vi "insertSoc_trans.vi"(8 "error in (no error)":errorcluster, 10 "input cluster":T3, 11 "connection reference":T1) -> (0 "error out":errorcluster, 3 "connection reference out":T1)   [LabVIEW 2012]
uses:
  <vilib>/addons/database/Connection.llb/Conn ObjectReference.ctl
  <vilib>/addons/database/NI_Database_API.lvlib
panel:
  in  "Cluster":T2
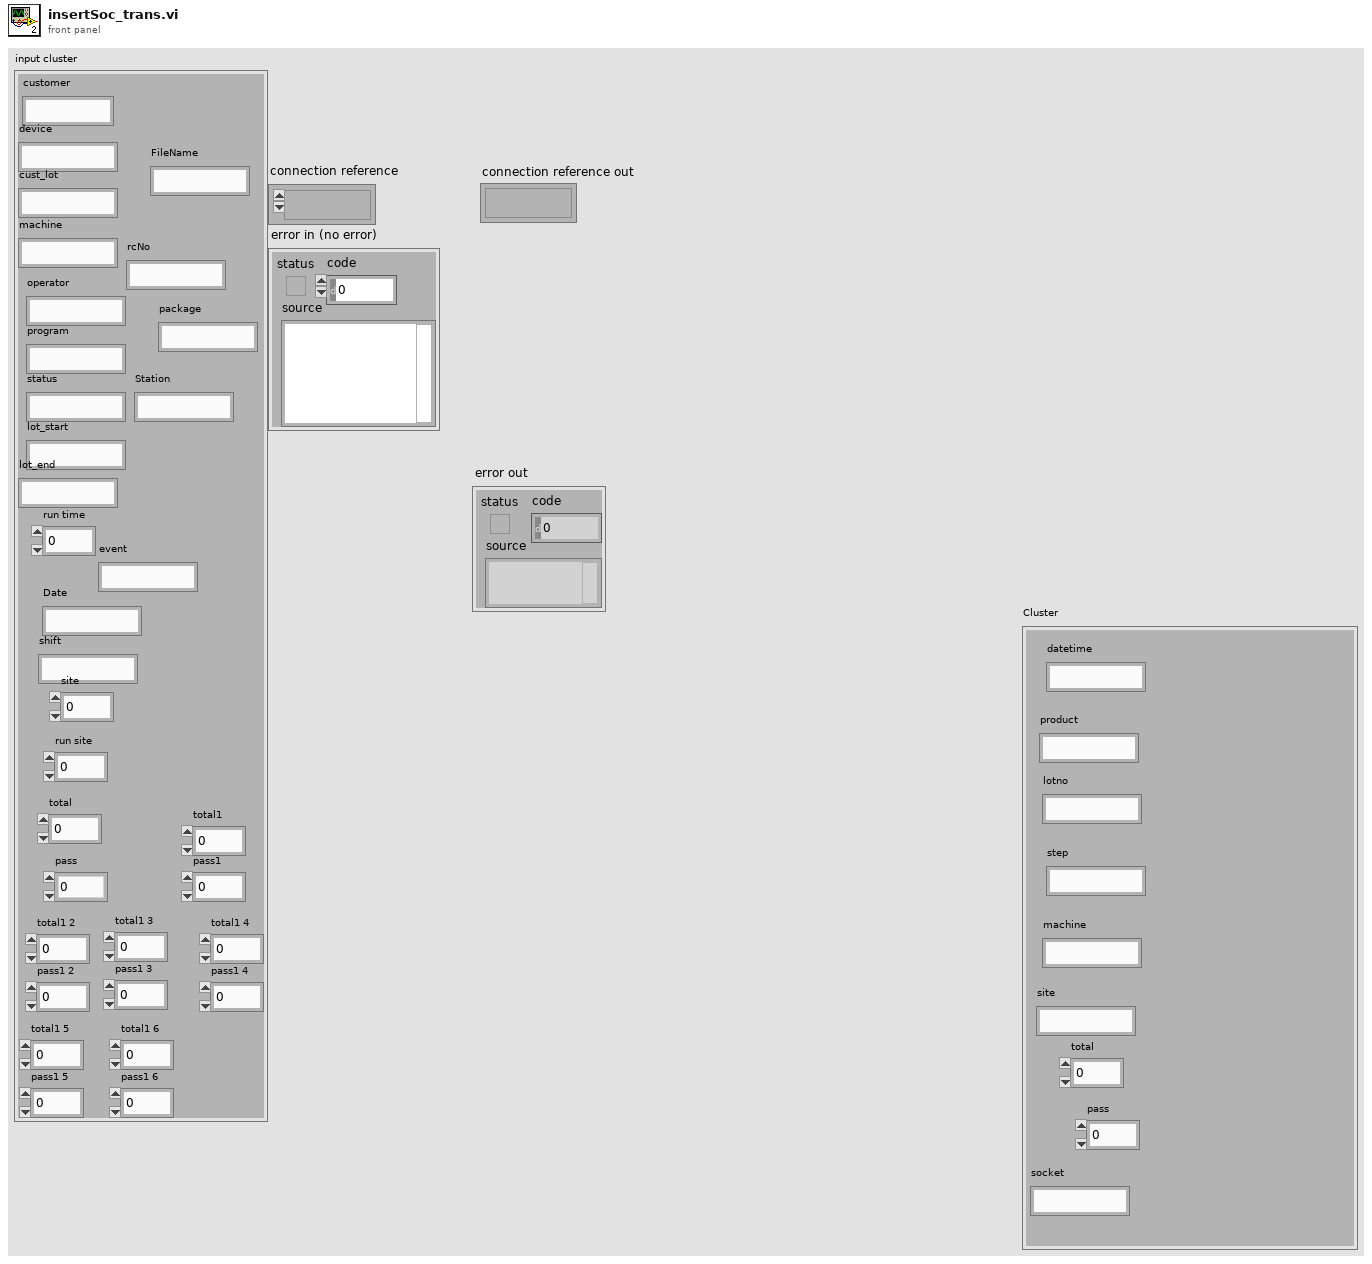
[diagram p1: front panel]
types:
  T1 = typedef "NI_Database_API.lvlib/Conn ObjectReference.ctl" = refnum<k1>
  T2 = cluster{"datetime":string, "product":string, "lotno":string, "step":string, "machine":string, "site":string, "total":dbl, "pass":dbl, "socket":string}
  T3 = cluster{"customer":string, "device":string, "FileName":string, "cust_lot":string, "machine":string, "rcNo":string, "package":string, "operator":string, "program":string, "status":string, "lot_start":string, "lot_end":string, "run time":dbl, "event":string, "Date":string, "shift":string, "site":dbl, "run site ":dbl, "total":dbl, "pass":dbl, "total1":dbl, "pass1":dbl, "total1 2":dbl, "pass1 2":dbl, "total1 3":dbl, "pass1 3":dbl, "total1 4":dbl, "pass1 4":dbl, "total1 5":dbl, "pass1 5":dbl, "total1 6":dbl, "pass1 6":dbl, "Station":string}
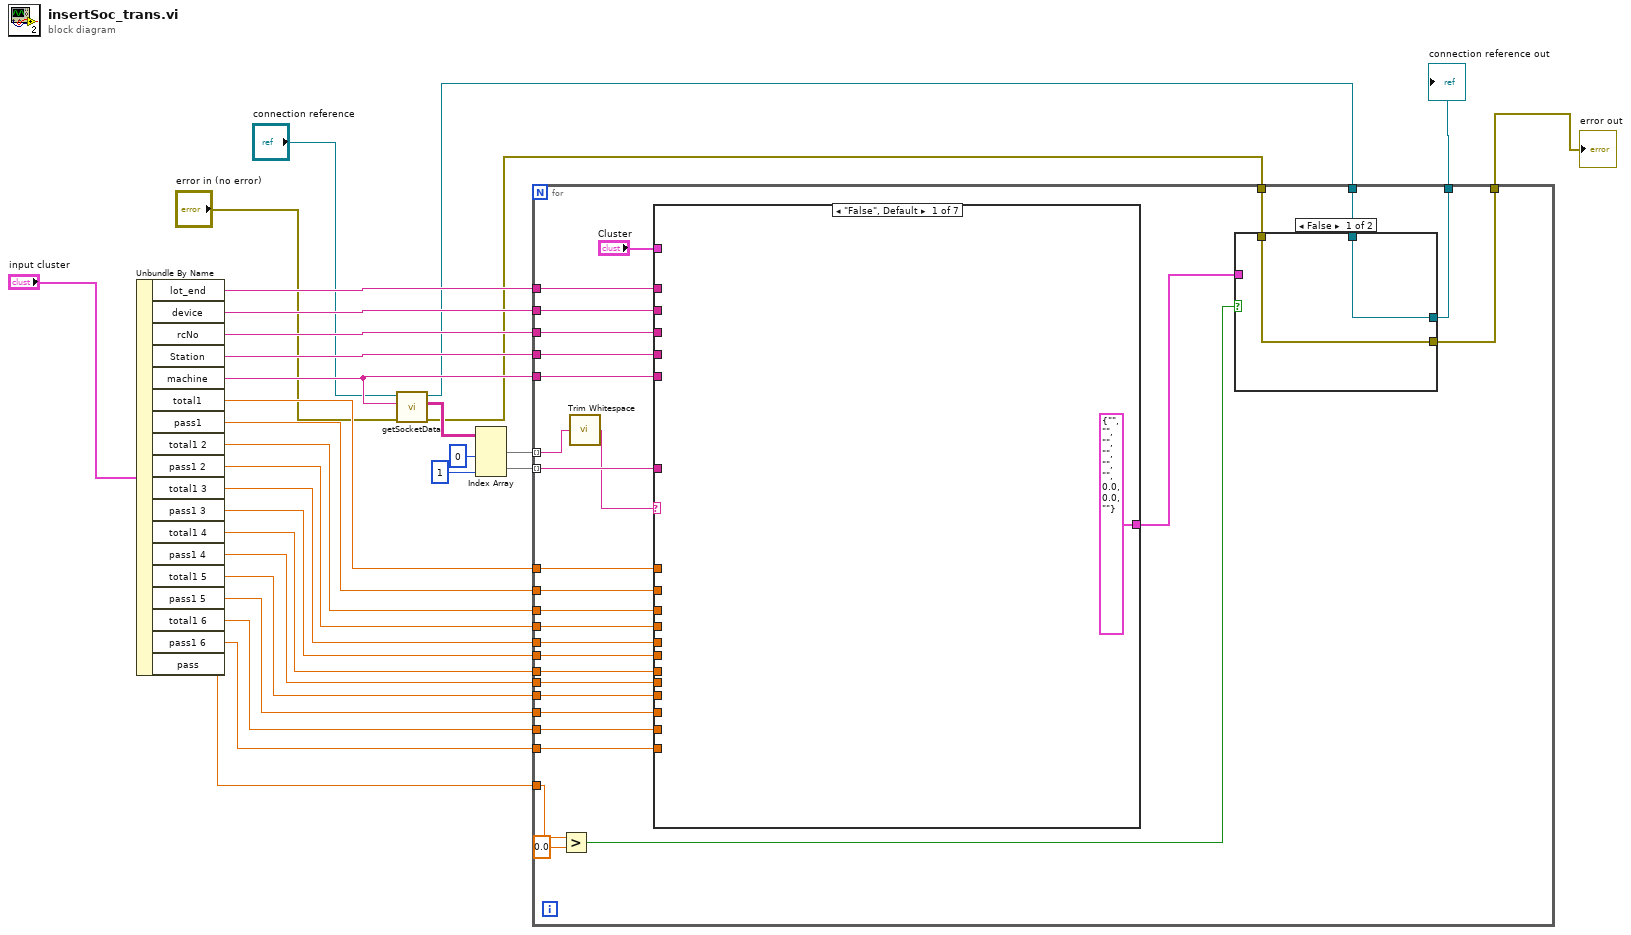
[diagram p0: block diagram]
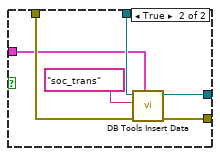
[diagram p2: hidden frame]
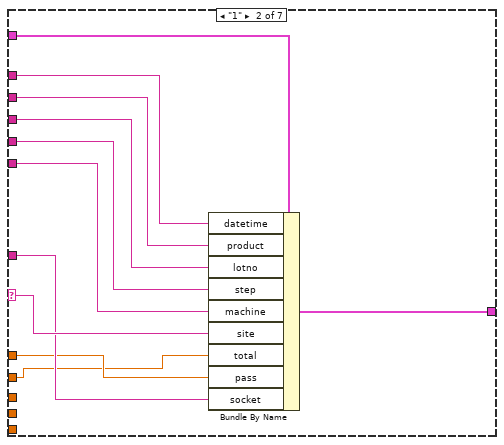
[diagram p3: hidden frame]
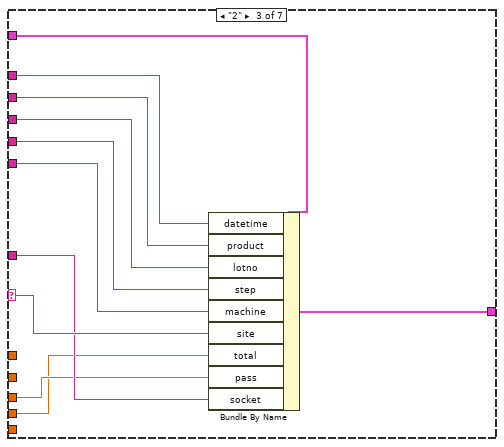
[diagram p4: hidden frame]
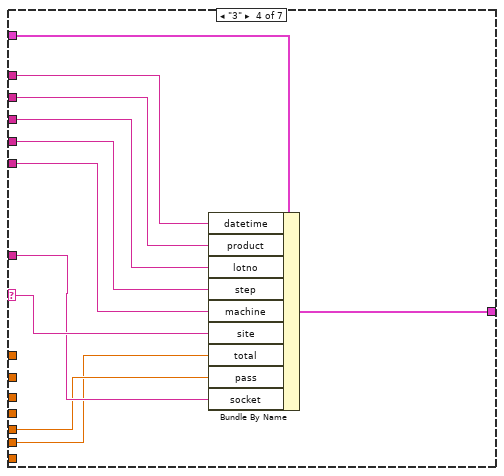
[diagram p5: hidden frame]
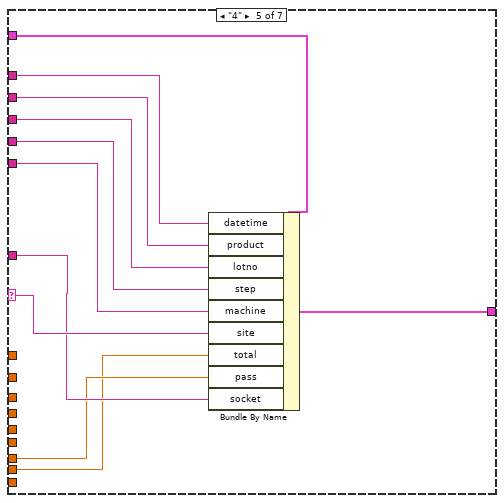
[diagram p6: hidden frame]
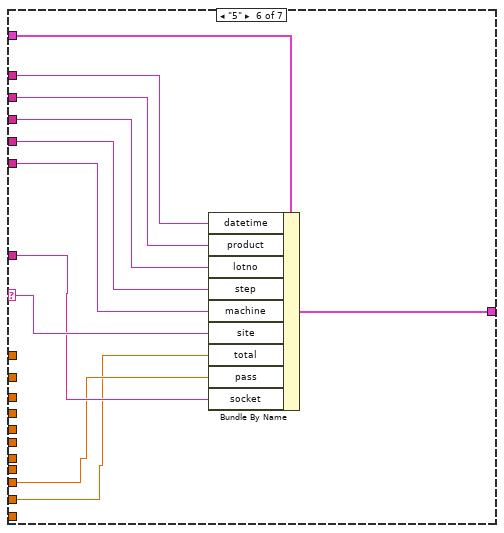
[diagram p7: hidden frame]
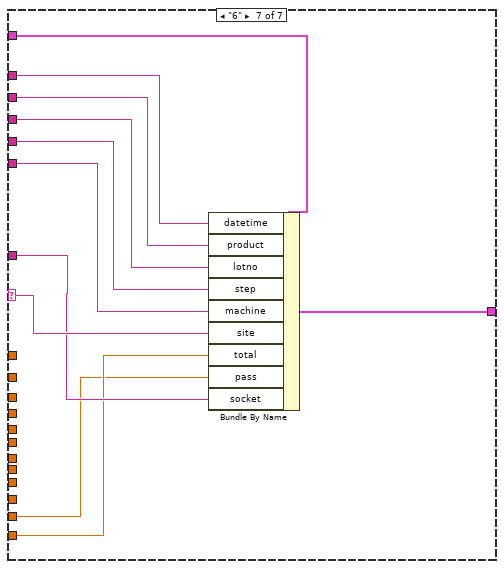
[diagram p8: hidden frame]
diagram:
  n1 = Unbundle By Name("input cluster") -> ("lot_end"=w24:string, "device"=w23:string, "rcNo"=w22:string, "Station"=w21:string, "machine"=w20:string, "total1"=w19:dbl, "pass1"=w18:dbl, "total1 2"=w17:dbl, "pass1 2"=w16:dbl, "total1 3"=w15:dbl, "pass1 3"=w14:dbl, "total1 4"=w13:dbl, "pass1 4"=w12:dbl, "total1 5"=w11:dbl, "pass1 5"=w10:dbl, "total1 6"=w9:dbl, "pass1 6"=w8:dbl, "pass"=w1:dbl)
  n2 = call "getSocketData.vi"("error in (no error)"="error in (no error)", "Machine"=w20, "connection reference"="connection reference") -> ("error out"=w4:errorcluster, "array"=w29:string[][], "connection reference 2"=w5:T1)  [unwired: 6 in]
  n3 = Index Array(array=w29, index (col) #1=0 ("disabled index (col)"), index (col) #2=1 ("index (col)")) -> (element #1=w26:string[], element #2=w25:string[])  [unwired: 2 in]
  n4 = for {
    tunnel: w26 -> [w36] mode=indexing
    tunnel: w25 -> [w48] mode=indexing
    tunnel: w24 -> [w59]
    tunnel: w23 -> [w58]
    tunnel: w22 -> [w57]
    tunnel: w21 -> [w56]
    tunnel: w20 -> [w55]
    tunnel: w19 -> [w54]
    tunnel: w18 -> [w53]
    tunnel: w17 -> [w52]
    tunnel: w16 -> [w51]
    tunnel: w15 -> [w50]
    tunnel: w14 -> [w49]
    tunnel: w13 -> [w47]
    tunnel: w12 -> [w46]
    tunnel: w11 -> [w45]
    tunnel: w10 -> [w44]
    tunnel: w9 -> [w43]
    tunnel: w8 -> [w42]
    tunnel: w5 -> [w41]
    tunnel: w4 -> [w40]
    tunnel: [w38] -> w2
    tunnel: [w37] -> w3
    tunnel: w1 -> [w33]
    n5 = Greater?(x=w33, y=0.0) -> (0:w31:bool)
    n6 = call <vilib>:"Trim Whitespace.vi"("string"=w36) -> ("trimmed string"=w35:string)  [unwired: 1 in]
    n7 = case shown="\"False\", Default" w35 {
      selector: w35 -> [_ w74 w85 w96 w107 w118 w129]
      tunnel: w59 -> [_ w79 w90 w101 w112 w123 w134]
      tunnel: w58 -> [_ w78 w89 w100 w111 w122 w133]
      tunnel: w57 -> [_ w77 w88 w99 w110 w121 w132]
      tunnel: w56 -> [_ w76 w87 w98 w109 w120 w131]
      tunnel: w55 -> [_ w75 w86 w97 w108 w119 w130]
      tunnel: w54 -> [_ w70 _ _ _ _ _]
      tunnel: w53 -> [_ w69 _ _ _ _ _]
      tunnel: w52 -> [_ _ w81 _ _ _ _]
      tunnel: w51 -> [_ _ w80 _ _ _ _]
      tunnel: w50 -> [_ _ _ w92 _ _ _]
      tunnel: w49 -> [_ _ _ w91 _ _ _]
      tunnel: w48 -> [_ w73 w84 w95 w106 w117 w128]
      tunnel: w47 -> [_ _ _ _ w103 _ _]
      tunnel: w46 -> [_ _ _ _ w102 _ _]
      tunnel: w45 -> [_ _ _ _ _ w114 _]
      tunnel: w44 -> [_ _ _ _ _ w113 _]
      tunnel: w43 -> [_ _ _ _ _ _ w124]
      tunnel: w42 -> [_ _ _ _ _ _ w125]
      tunnel: [T2 {"datetime"="", "product"="", "lotno"="", "step"="", "machine"="", "site"="", "total"=0.0, "pass"=0.0, "socket"=""} ("Cluster") w72 w83 w94 w105 w116 w127] -> w39
      tunnel: "Cluster" -> [_ w71 w82 w93 w104 w115 w126]
      frame "False", Default {
      }
      frame "1" {
        n8 = Bundle By Name(cluster=w71, "datetime"=w79, "product"=w78, "lotno"=w77, "step"=w76, "machine"=w75, "site"=w74, "total"=w69, "pass"=w70, "socket"=w73) -> (w72:T2)
      }
      frame "2" {
        n9 = Bundle By Name(cluster=w82, "datetime"=w90, "product"=w89, "lotno"=w88, "step"=w87, "machine"=w86, "site"=w85, "total"=w80, "pass"=w81, "socket"=w84) -> (w83:T2)
      }
      frame "3" {
        n10 = Bundle By Name(cluster=w93, "datetime"=w101, "product"=w100, "lotno"=w99, "step"=w98, "machine"=w97, "site"=w96, "total"=w91, "pass"=w92, "socket"=w95) -> (w94:T2)
      }
      frame "4" {
        n11 = Bundle By Name(cluster=w104, "datetime"=w112, "product"=w111, "lotno"=w110, "step"=w109, "machine"=w108, "site"=w107, "total"=w102, "pass"=w103, "socket"=w106) -> (w105:T2)
      }
      frame "5" {
        n12 = Bundle By Name(cluster=w115, "datetime"=w123, "product"=w122, "lotno"=w121, "step"=w120, "machine"=w119, "site"=w118, "total"=w113, "pass"=w114, "socket"=w117) -> (w116:T2)
      }
      frame "6" {
        n13 = Bundle By Name(cluster=w126, "datetime"=w134, "product"=w133, "lotno"=w132, "step"=w131, "machine"=w130, "site"=w129, "total"=w125, "pass"=w124, "socket"=w128) -> (w127:T2)
      }
    }
    n14 = case shown="False" w31 {
      tunnel: w41 -> [w61 w67]
      tunnel: w40 -> [w60 w66]
      tunnel: w39 -> [_ w64]
      tunnel: [w61 w63] -> w38
      tunnel: [w60 w62] -> w37
      frame False {
      }
      frame True {
        n15 = call <vilib>:"DB Tools Insert Data.vi"("data"=w64, "error in (no error)"=w66, "table"="soc_trans", "connection reference"=w67) -> ("error out"=w62:errorcluster, "connection reference out"=w63:T1)  [unwired: 6 in]
      }
    }
  }
  "error out" <- w3
  "connection reference out" <- w2
